vi "Get_link_info.vi"(0 "VI Name":string) -> (1 "Server IP & Port":string, 2 "Path name":path, 3 "Application reference":refnum<vi>, 4 "Local Call?":bool)   [LabVIEW 2016]
uses:
  Anemometry/Anemometry Sub Vis/Controls/Serveds.ctl
  Anemometry/Anemometry Sub Vis/Controls/App_Global.ctl
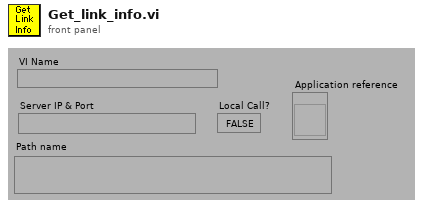
[diagram p1: front panel]
types:
  T1 = typedef "App_Global.ctl" = enum16{"Read Global", "Write to Global", "Initialise Array"}
  T2 = typedef "Serveds.ctl" = enum16{"Read Global", "Load Global From File"}
  T3 = typedef "App_Ref_Cluster.ctl" = cluster{"Server IP & Port No":string, "Application reference":refnum<vi>}
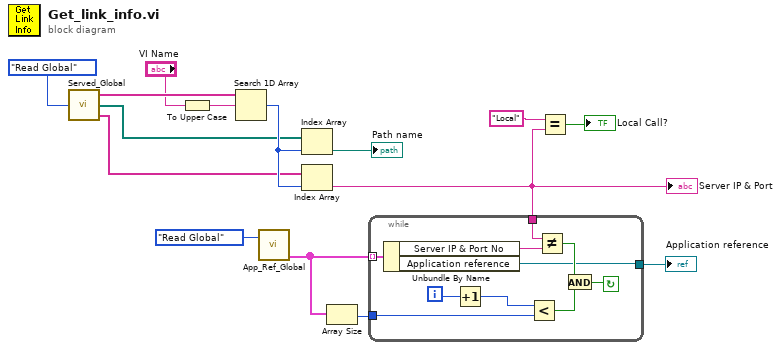
[diagram p0: block diagram]
diagram:
  n1 = call "Served_Global.vi"("Mode"=Serveds."Read Global") -> ("Served VI Name"=w12:string[], "Served VI Path"=w10:path[], "Served IP Number & Port No"=w11:string[])
  n2 = To Upper Case(1:"VI Name") -> (0:w6:string)
  n3 = Search 1D Array(1D array=w12, element=w6) -> (index of element=w15:i32)  [unwired: 1 out]
  n4 = call "App_Ref_Global.vi"("Mode"=App_Global."Read Global") -> ("Output Array"=w4:T3[])  [unwired: 1 in, 1 out]
  n5 = Index Array(array=w10, index=w15) -> (element=→"Path name":path)
  n6 = Index Array(array=w11, index=w15) -> (element=w1:string)
  "Server IP & Port" <- w1
  n7 = Array Size(array=w4) -> (size(s)=w3:i32)
  n8 = while {
    tunnel: [w16] -> w2
    tunnel: w3 -> [w21]
    tunnel: w1 -> [w23]
    tunnel: w4 -> [w25] mode=indexing
    i -> [w22]
    stop <- w17 continue-if-true
    n9 = Unbundle By Name(w25) -> ("Server IP & Port No"=w24:string, "Application reference"=w16:refnum<vi>)
    n10 = Increment(x=w22) -> (x+1=w20:i32)
    n11 = Less?(x=w20, y=w21) -> (x < y?=w19:bool)
    n12 = Not Equal?(x=w23, y=w24) -> (x != y?=w18:bool)
    n13 = And(x=w18, y=w19) -> (x .and. y?=w17:bool)
  }
  "Application reference" <- w2
  n14 = Equal?(x="Local" ("t"), y=w1) -> (x = y?=→"Local Call?":bool)
